vi "Read Services.vi"(8 "error in (no error)":errorcluster, 10 "Wash Car Cost":T1(array[cluster]) {"Cost" format="$ %.1f"}, 11 "Paquetes Disponibles in":refnum<class "Paquetes Disponibles.lvclass">) -> (0 "error out":errorcluster, 3 "Paquetes Disponibles out":refnum<class "Paquetes Disponibles.lvclass">)   [LabVIEW 2020, in "Paquetes Disponibles.lvlib" / "Paquetes Disponibles.lvclass"]
uses:
  Paquetes Disponibles.lvclass
  Paquetes Disponibles.lvclass/Paquetes Disponibles.ctl
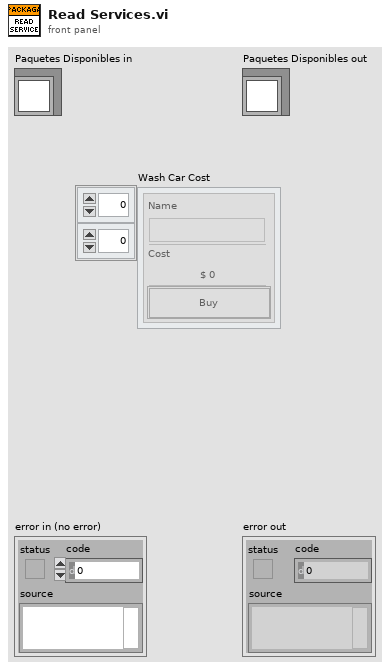
[diagram p1: front panel]
types:
  T1 = cluster{"Name":string, "Cost":u8, "Comprar":bool}[][]
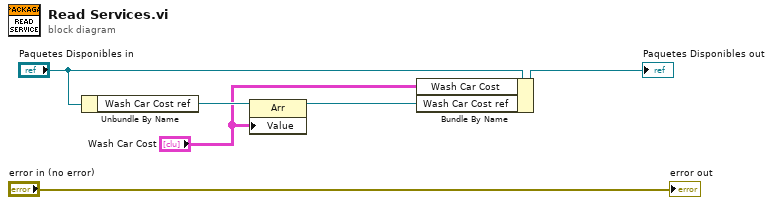
[diagram p0: block diagram]
diagram:
  n1 = Unbundle By Name("Paquetes Disponibles in") -> ("Wash Car Cost ref"=w2:refnum<vi>)
  n2 = property class="Arr"(reference=w2, "Value"="Wash Car Cost") -> (reference out=w3:refnum<vi>)  [unwired: 1 in, 1 out]
  n3 = Bundle By Name(cluster="Paquetes Disponibles in", "Wash Car Cost"="Wash Car Cost", "Wash Car Cost ref"=w3) -> (→"Paquetes Disponibles out":refnum<class "Paquetes Disponibles.lvclass">)
  "error out" <- "error in (no error)"
